vi "test Boolean Data Integrity.vi"(8 "error in (no error)":errorcluster, 11 "Data Manipulation Tests in":refnum<class "Data Manipulation Tests.lvclass">) -> (0 "error out":errorcluster, 3 "Data Manipulation Tests out":refnum<class "Data Manipulation Tests.lvclass">)   [LabVIEW 2017, in "Pointer Tests.lvlib" / "Data Manipulation Tests.lvclass"]
uses:
  Data Manipulation Tests.lvclass
  Source/Classes/Pointer/Pointer.lvclass/Pointer.ctl
  Source/Classes/Pointer/Public/New/New (1B).vi
  Source/Classes/Pointer/Public/Write/Write (0D Bool).vi
  Source/Classes/Pointer/Public/New/New (4B).vi
  Source/Classes/Pointer/Public/Write/Write (1D Bool).vi
  Source/Classes/Pointer/Private/Allocate.vi
  Source/Classes/Pointer/Public/Write (No Check)/Write (No Check 0D Bool).vi
  Source/Classes/Pointer/Protected/Parameter Checking/Check Null Pointer.vi
  Source/Classes/Pointer/Protected/Parameter Checking/Check Subset.vi
  Source/Classes/Pointer/Private/Deallocate.vi
  Source/Classes/Pointer/Public/Write (No Check)/Write (No Check 1D Bool).vi
  Source/Classes/Pointer/Protected/Parameter Checking/Check Subset (Power of 2).vi
  Source/Classes/Pointer/API/Accessors/Set Address.vi
  Source/Classes/Pointer/API/Accessors/Set Size.vi
  Source/Classes/Pointer/Private/Set Internal.vi
  Source/Classes/Pointer/API/Accessors/Get Address.vi
  Source/Classes/Pointer/Protected/Errors.vi
  Source/Classes/Pointer/Protected/Error VIs/Null Pointer.vi
  Source/Classes/Pointer/Protected/Error VIs/Out of Bounds.vi
  Source/Classes/Pointer/API/Accessors/Get Size.vi
  Source/Classes/Pointer/Protected/Get Internal.vi
  Source/Classes/Pointer/Protected/Error VIs/Zone.vi
  Source/Classes/Pointer/Private/Count to Size.vi
  Source/Classes/Pointer/Protected/Error Building/Create Error.vi
  Source/VIs/Write String into Source.vi
  Source/Classes/Pointer/Protected/Error Building/Write Pointer Size.vi
  Source/VIs/Write Number into Source.vi
  Source/VIs/VIs for Poly/Write U64 into Source.vi
  Source/Constants/Constants.vi
  Source/Constants/Library Name.vi
  Source/Classes/Pointer/Protected/Error Building/Get Error Info.vi
  Source/VIs/Create Error Cluster.vi
  Source/VIs/VIs for Poly/Create Error Cluster (256B).vi
  Source/VIs/Set Error Status.vi
  Source/VIs/Set Error Code.vi
  Source/VIs/Set Error Source.vi
  Source/Classes/Pointer/Pointer.lvclass
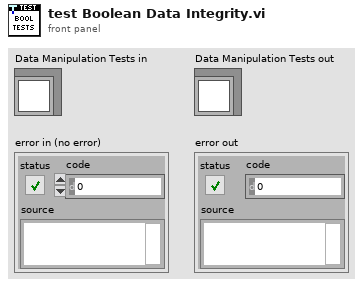
[diagram p1: front panel]
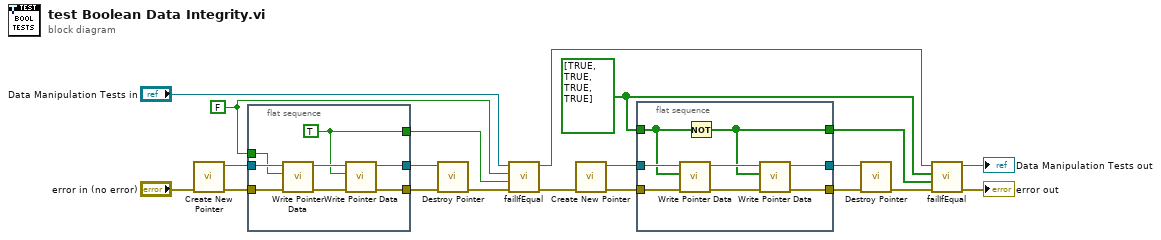
[diagram p0: block diagram]
diagram:
  w14 = bool[] [TRUE, TRUE, TRUE, TRUE] ("value")
  w7 = FALSE ("value")
  n1 = call-poly "Create New Pointer.vi"("error in (no error)"="error in (no error)") -> ("error out"=w4:errorcluster, "Pointer"=w1:refnum<class "Pointer.lvclass">)  [unwired: 9 in]
  n2 = flat-sequence {
    tunnel: w1 -> [w28]
    tunnel: [w26] -> w2
    tunnel: [w25] -> w3
    tunnel: w4 -> [w23]
    tunnel: w7 -> [w22]
    tunnel: [w21] -> w8
    frame #0 {
      w21 = TRUE ("value")
      n3 = call-poly "Write Pointer Data.vi"("error in (no error)"=w23, "value"=w22, "Pointer in"=w28) -> ("error out"=w24:errorcluster, "Pointer out"=w27:refnum<class "Pointer.lvclass">)  [unwired: 5 in, 2 out]
      n4 = call-poly "Write Pointer Data.vi"("error in (no error)"=w24, "value"=w21, "Pointer in"=w27) -> ("error out"=w25:errorcluster, "Pointer out"=w26:refnum<class "Pointer.lvclass">)  [unwired: 5 in, 2 out]
    }
  }
  n5 = call "Destroy Pointer.vi"("error in (no error)"=w3, "Pointer in"=w2) -> ("error out"=w5:errorcluster)  [unwired: 8 in, 1 out]
  n6 = call-dynamic "failIfEqual.vi"("error in (no error)"=w5, "y"=w8, "x"=w7, "TestCase in"="Data Manipulation Tests in") -> ("error out"=w18:errorcluster, "TestCase out"=w17:refnum<class "Data Manipulation Tests.lvclass">)  [unwired: 6 in]
  n7 = call-poly "Create New Pointer.vi"("error in (no error)"=w18) -> ("error out"=w12:errorcluster, "Pointer"=w9:refnum<class "Pointer.lvclass">)  [unwired: 9 in]
  n8 = flat-sequence {
    tunnel: w9 -> [w36]
    tunnel: [w34] -> w10
    tunnel: [w33] -> w11
    tunnel: w12 -> [w31]
    tunnel: w14 -> [w30]
    tunnel: [w29] -> w15
    frame #0 {
      n9 = call-poly "Write Pointer Data.vi"("error in (no error)"=w31, "buffer in"=w30, "Pointer in"=w36) -> ("error out"=w32:errorcluster, "Pointer out"=w35:refnum<class "Pointer.lvclass">)  [unwired: 5 in, 2 out]
      n10 = Not(x=w30) -> (.not. x?=w29:bool[])
      n11 = call-poly "Write Pointer Data.vi"("error in (no error)"=w32, "buffer in"=w29, "Pointer in"=w35) -> ("error out"=w33:errorcluster, "Pointer out"=w34:refnum<class "Pointer.lvclass">)  [unwired: 5 in, 2 out]
    }
  }
  n12 = call "Destroy Pointer.vi"("error in (no error)"=w11, "Pointer in"=w10) -> ("error out"=w13:errorcluster)  [unwired: 8 in, 1 out]
  n13 = call-dynamic "failIfEqual.vi"("error in (no error)"=w13, "y"=w15, "x"=w14, "TestCase in"=w17) -> ("error out"=→"error out":errorcluster, "TestCase out"=→"Data Manipulation Tests out":refnum<class "Data Manipulation Tests.lvclass">)  [unwired: 6 in]
